vi "frf2mag-phase.vi"(10 "G_frf":cdb[](array[numeric])) -> (0 "phase [deg]":dbl[](array[numeric]), 3 "mag-dB":dbl[](array[numeric]))   [LabVIEW 2017]
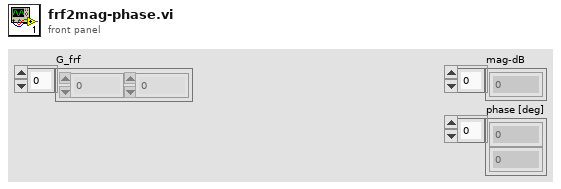
[diagram p1: front panel]
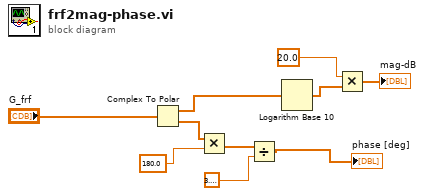
[diagram p0: block diagram]
diagram:
  n1 = Complex To Polar(r * e^(i*theta)="G_frf") -> (r=w2:dbl[], theta=w10:dbl[])
  n2 = Multiply(x=w10, y=180.0) -> (x*y=w8:dbl[])
  n3 = Divide(x=w8, y=3.141592653589793) -> (x/y=→"phase [deg]":dbl[])
  n4 = Logarithm Base 10(1:w2) -> (0:w6:dbl[])
  n5 = Multiply(x=20.0, y=w6) -> (x*y=→"mag-dB":dbl[])
